vi "deleteDetails.vi"(8 "error in (no error)":errorcluster, 10 "details":T2, 11 "reference in":refnum<class "Devices Controller.lvclass">) -> (0 "error out":errorcluster, 3 "reference out":refnum<class "Devices Controller.lvclass">)   [LabVIEW 2015, in "Devices Controller.lvclass"]
uses:
  Devices Controller.lvclass
  deviceType.ctl
  APP/excelFile_class/fileType.ctl
  APP/k4b2_class/k4b2.lvclass
  APP/fitmate_class/fitmate.lvclass
  APP/cpet_class/cpet.lvclass
  APP/rmr_class/rmr.lvclass
  APP/bb-pft_class/bb-pft.lvclass
  APP/bodpod_class/bodpod.lvclass
  APP/peapod_class/peapod.lvclass
  APP/k5_class/k5.lvclass
  APP/excelFile_class/excelFile.lvclass
  File Controller_llb/File Controller.lvclass
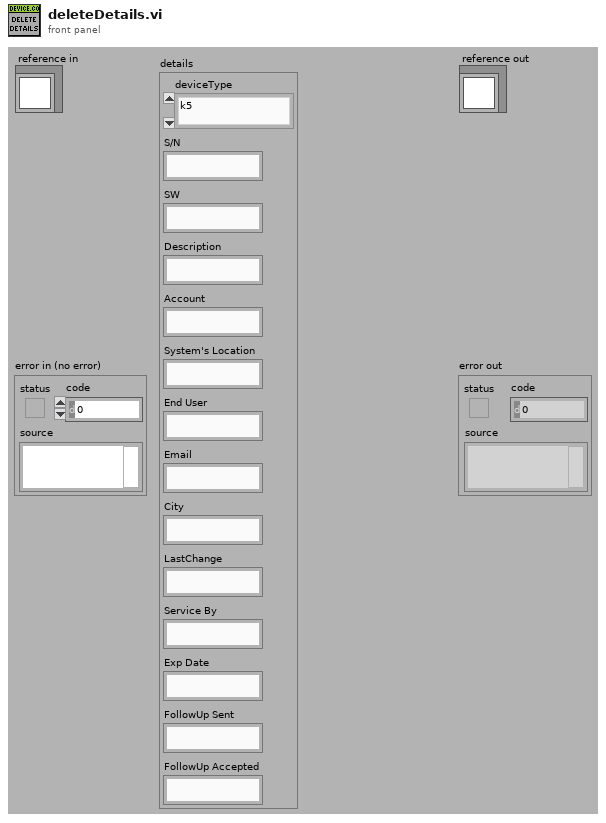
[diagram p1: front panel]
types:
  T1 = typedef "Devices Controller.lvclass/deviceType.ctl" = enum16{"k5", "k4b2", "fitmate", "cpet", "rmr", "bodyBoxPft", "bp", "pp"}
  T2 = cluster{"deviceType":T1, "S/N":string, "SW":string, "Description":string, "Account":string, "System's Location":string, "End User":string, "Email":string, "City":string, "LastChange":string, "Service By":string, "Exp Date":string, "FollowUp Sent":string, "FollowUp Accepted":string}
  T3 = typedef "excelFile.lvclass/fileType.ctl" = enum16{"devices", "items", "partsTracking", "TSR"}
  T4 = typedef "Devices Controller.lvclass/ObjectAttributesRef.ctl" = refnum<data-value>
  T5 = typedef "Devices Controller.lvclass/ObjectAttributes.ctl" = cluster{"MyAttribute":dbl, "file_controller_ref":refnum<class "File Controller.lvclass">, "data":string[][][], "devices_refs":cluster{"k4b2_refs":refnum<class "k4b2.lvclass">[], "rmr_refs":refnum<class "rmr.lvclass">[], "bod_pod_refs":refnum<class "bodpod.lvclass">[], "cpet_refs":refnum<class "cpet.lvclass">[], "fitmate_refs":refnum<class "fitmate.lvclass">[], "pea_pod_refs":refnum<class "peapod.lvclass">[], "k5_refs":refnum<class "k5.lvclass">[], "bb-pft_refs":refnum<class "bb-pft.lvclass">[]}}
  T6 = cluster{"k4b2_refs":refnum<class "k4b2.lvclass">[], "rmr_refs":refnum<class "rmr.lvclass">[], "bod_pod_refs":refnum<class "bodpod.lvclass">[], "cpet_refs":refnum<class "cpet.lvclass">[], "fitmate_refs":refnum<class "fitmate.lvclass">[], "pea_pod_refs":refnum<class "peapod.lvclass">[], "k5_refs":refnum<class "k5.lvclass">[], "bb-pft_refs":refnum<class "bb-pft.lvclass">[]}
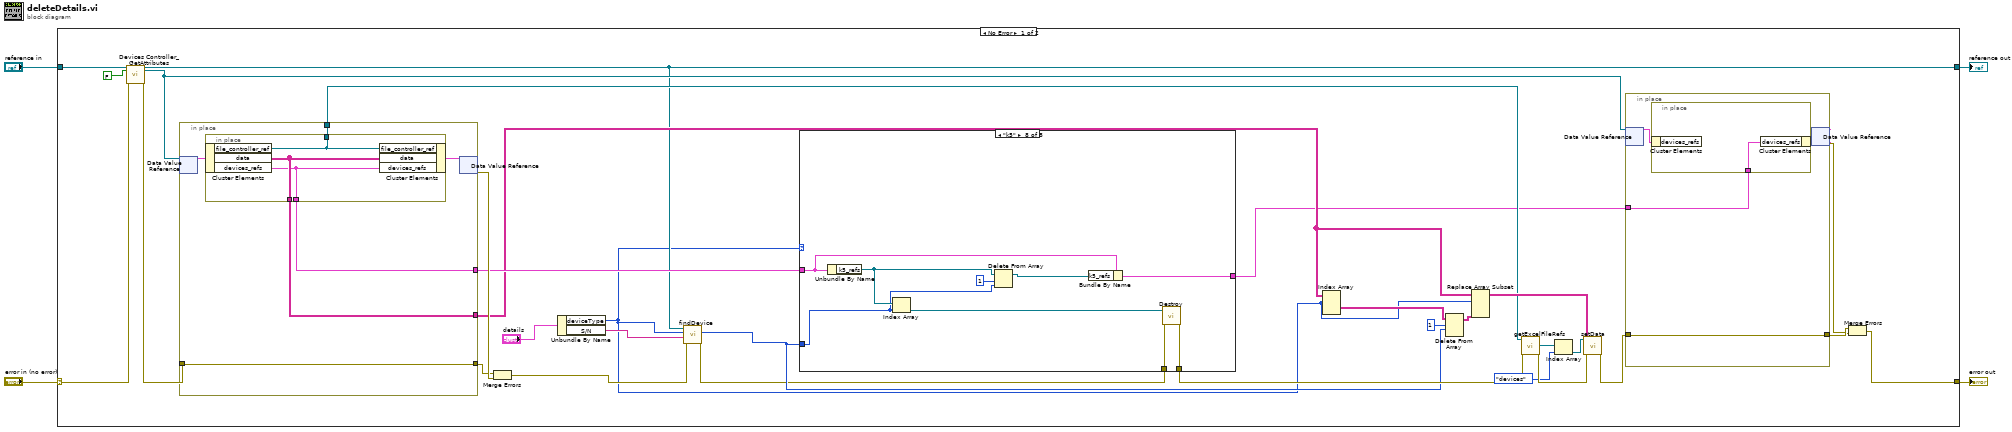
[diagram p0: block diagram]
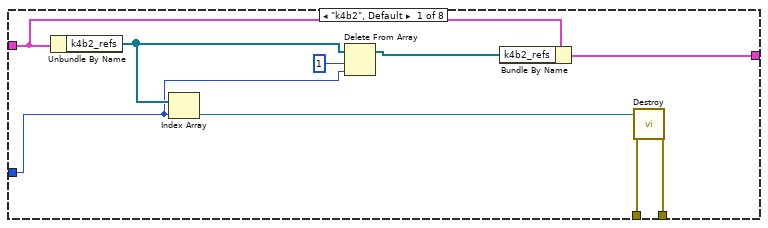
[diagram p2: hidden frame]
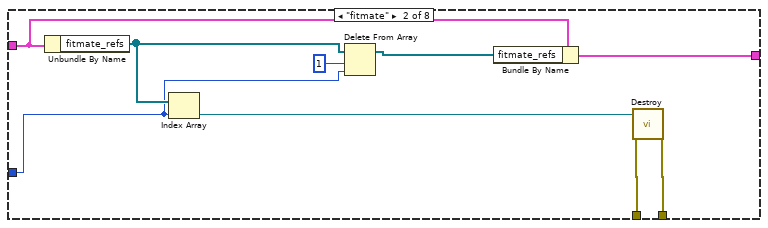
[diagram p3: hidden frame]
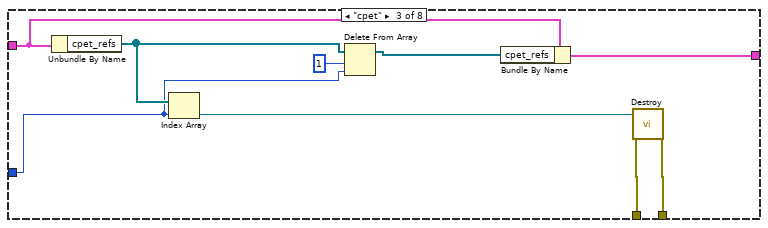
[diagram p4: hidden frame]
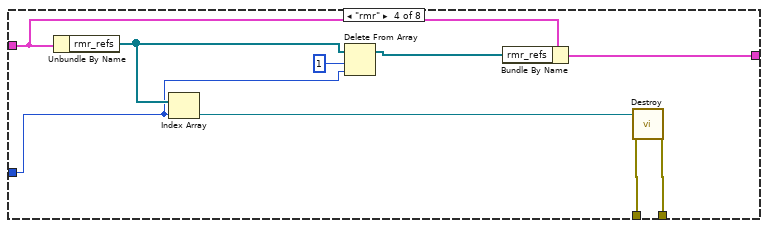
[diagram p5: hidden frame]
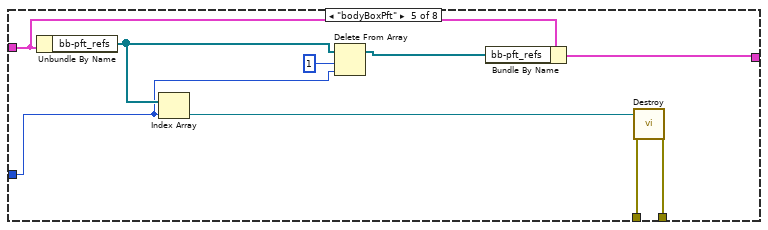
[diagram p6: hidden frame]
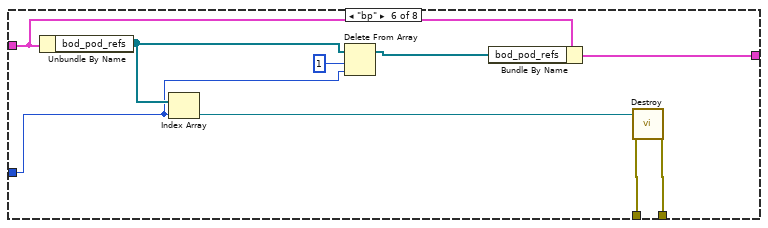
[diagram p7: hidden frame]
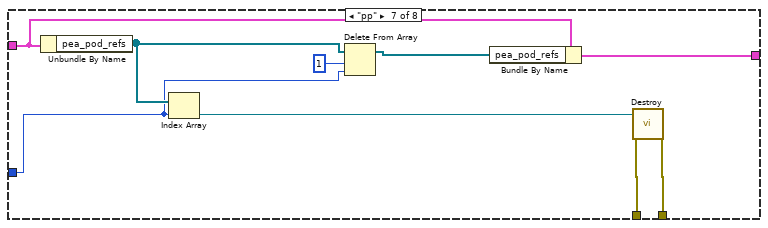
[diagram p8: hidden frame]
diagram:
  n1 = case shown="No Error" "error in (no error)" {
    selector: "error in (no error)" -> [w31 w123]
    tunnel: [w11 w123] -> w3
    tunnel: [w10 w122] -> w1
    tunnel: "reference in" -> [w33 w122]
    frame No Error {
      n2 = call "Devices Controller_GetAttributes.vi"("reference in"=w33, "return data? (T)"=FALSE, "error in (no error)"=w31) -> ("reference out"=w10:refnum<class "Devices Controller.lvclass">, "attributes ref"=w14:T4, "error out"=w30:errorcluster)  [unwired: 13 in, 1 out]
      n3 = in-place {
        in-place-border: w30 -> [w116]
        in-place-border: [w116] -> w34
        in-place-border: [w115] -> w20
        in-place-border: [w114] -> w29
        in-place-border: [w113] -> w19
        n4 = in-place-dvr #1(w14) -> (w117:T5)  [unwired: 1 out]
        n5 = in-place {
          in-place-border: [w121] -> w115
          in-place-border: [w120] -> w114
          in-place-border: [w119] -> w113
          n6 = in-place-cluster #2(w117) -> ("file_controller_ref"=w119:refnum<class "File Controller.lvclass">, "data"=w121:string[][][], "devices_refs"=w120:T6)
          n7 = in-place-cluster #2("file_controller_ref"=w119, "data"=w121, "devices_refs"=w120) -> (w118:T5)
        }
        n8 = in-place-dvr #1(w118) -> (w35:errorcluster)  [unwired: 1 out]
      }
      n9 = Merge Errors(w34, w35) -> (w8:errorcluster)
      n10 = Unbundle By Name("details") -> ("deviceType"=w5:T1, "S/N"=w6:string)
      n11 = call "findDevice.vi"("error in (no error)"=w8, "S/N:"=w6, "Device Type:"=w5, "reference in"=w10) -> ("error out"=w7:errorcluster, "index of element"=w9:i32)  [unwired: 4 in, 2 out]
      n12 = case shown="\"k5\"" w5 {
        tunnel: w29 -> [w43 w52 w61 w70 w81 w88 w97 w109]
        tunnel: w9 -> [w44 w53 w62 w71 w80 w89 w98 w108]
        tunnel: w7 -> [w49 w58 w67 w76 w78 w94 w103 w105]
        tunnel: [w48 w57 w66 w75 w77 w93 w102 w104] -> w21
        tunnel: [w41 w50 w59 w68 w79 w86 w95 w106] -> w15
        frame "k4b2", Default {
          n13 = Unbundle By Name(w43) -> ("k4b2_refs"=w45:refnum<class "k4b2.lvclass">[])
          n14 = Index Array(array=w45, index=w44) -> (element=w47:refnum<class "k4b2.lvclass">)
          n15 = Delete From Array(array=w45, length=1, index=w44) -> (array with subset deleted=w42:refnum<class "k4b2.lvclass">[])  [unwired: 1 out]
          n16 = Bundle By Name(cluster=w43, "k4b2_refs"=w42) -> (w41:T6)
          n17 = call-dynamic "Destroy.vi"("reference in"=w47, "error in (no error)"=w49) -> ("error out"=w48:errorcluster)  [unwired: 16 in, 1 out]
        }
        frame "fitmate" {
          n18 = Unbundle By Name(w52) -> ("fitmate_refs"=w54:refnum<class "fitmate.lvclass">[])
          n19 = Index Array(array=w54, index=w53) -> (element=w56:refnum<class "fitmate.lvclass">)
          n20 = Delete From Array(array=w54, length=1, index=w53) -> (array with subset deleted=w51:refnum<class "fitmate.lvclass">[])  [unwired: 1 out]
          n21 = Bundle By Name(cluster=w52, "fitmate_refs"=w51) -> (w50:T6)
          n22 = call-dynamic "Destroy.vi"("reference in"=w56, "error in (no error)"=w58) -> ("error out"=w57:errorcluster)  [unwired: 16 in, 1 out]
        }
        frame "cpet" {
          n23 = Unbundle By Name(w61) -> ("cpet_refs"=w63:refnum<class "cpet.lvclass">[])
          n24 = Index Array(array=w63, index=w62) -> (element=w65:refnum<class "cpet.lvclass">)
          n25 = Delete From Array(array=w63, length=1, index=w62) -> (array with subset deleted=w60:refnum<class "cpet.lvclass">[])  [unwired: 1 out]
          n26 = Bundle By Name(cluster=w61, "cpet_refs"=w60) -> (w59:T6)
          n27 = call-dynamic "Destroy.vi"("reference in"=w65, "error in (no error)"=w67) -> ("error out"=w66:errorcluster)  [unwired: 16 in, 1 out]
        }
        frame "rmr" {
          n28 = Unbundle By Name(w70) -> ("rmr_refs"=w72:refnum<class "rmr.lvclass">[])
          n29 = Index Array(array=w72, index=w71) -> (element=w74:refnum<class "rmr.lvclass">)
          n30 = Delete From Array(array=w72, length=1, index=w71) -> (array with subset deleted=w69:refnum<class "rmr.lvclass">[])  [unwired: 1 out]
          n31 = Bundle By Name(cluster=w70, "rmr_refs"=w69) -> (w68:T6)
          n32 = call-dynamic "Destroy.vi"("reference in"=w74, "error in (no error)"=w76) -> ("error out"=w75:errorcluster)  [unwired: 16 in, 1 out]
        }
        frame "bodyBoxPft" {
          n33 = Unbundle By Name(w81) -> ("bb-pft_refs"=w83:refnum<class "bb-pft.lvclass">[])
          n34 = Index Array(array=w83, index=w80) -> (element=w85:refnum<class "bb-pft.lvclass">)
          n35 = Delete From Array(array=w83, length=1, index=w80) -> (array with subset deleted=w82:refnum<class "bb-pft.lvclass">[])  [unwired: 1 out]
          n36 = Bundle By Name(cluster=w81, "bb-pft_refs"=w82) -> (w79:T6)
          n37 = call-dynamic "Destroy.vi"("reference in"=w85, "error in (no error)"=w78) -> ("error out"=w77:errorcluster)  [unwired: 16 in, 1 out]
        }
        frame "bp" {
          n38 = Unbundle By Name(w88) -> ("bod_pod_refs"=w90:refnum<class "bodpod.lvclass">[])
          n39 = Index Array(array=w90, index=w89) -> (element=w92:refnum<class "bodpod.lvclass">)
          n40 = Delete From Array(array=w90, length=1, index=w89) -> (array with subset deleted=w87:refnum<class "bodpod.lvclass">[])  [unwired: 1 out]
          n41 = Bundle By Name(cluster=w88, "bod_pod_refs"=w87) -> (w86:T6)
          n42 = call-dynamic "Destroy.vi"("reference in"=w92, "error in (no error)"=w94) -> ("error out"=w93:errorcluster)  [unwired: 16 in, 1 out]
        }
        frame "pp" {
          n43 = Unbundle By Name(w97) -> ("pea_pod_refs"=w99:refnum<class "peapod.lvclass">[])
          n44 = Index Array(array=w99, index=w98) -> (element=w101:refnum<class "peapod.lvclass">)
          n45 = Delete From Array(array=w99, length=1, index=w98) -> (array with subset deleted=w96:refnum<class "peapod.lvclass">[])  [unwired: 1 out]
          n46 = Bundle By Name(cluster=w97, "pea_pod_refs"=w96) -> (w95:T6)
          n47 = call-dynamic "Destroy.vi"("reference in"=w101, "error in (no error)"=w103) -> ("error out"=w102:errorcluster)  [unwired: 16 in, 1 out]
        }
        frame "k5" {
          n48 = Unbundle By Name(w109) -> ("k5_refs"=w110:refnum<class "k5.lvclass">[])
          n49 = Index Array(array=w110, index=w108) -> (element=w112:refnum<class "k5.lvclass">)
          n50 = Delete From Array(array=w110, length=1, index=w108) -> (array with subset deleted=w107:refnum<class "k5.lvclass">[])  [unwired: 1 out]
          n51 = Bundle By Name(cluster=w109, "k5_refs"=w107) -> (w106:T6)
          n52 = call-dynamic "Destroy.vi"("reference in"=w112, "error in (no error)"=w105) -> ("error out"=w104:errorcluster)  [unwired: 16 in, 1 out]
        }
      }
      n53 = Index Array(array=w20, index (dim 0)=w5) -> (element=w28:string[][])  [unwired: 2 in]
      n54 = Delete From Array(array=w28, length=1, index (row)=w9) -> (array with subset deleted=w27:string[][])  [unwired: 1 in, 1 out]
      n55 = Replace Array Subset(array=w20, new element=w27, index (dim 0)=w5) -> (w26:string[][][])  [unwired: 2 in]
      n56 = call "getExcelFileRefs.vi"("error in (no error)"=w21, "reference in"=w19) -> ("error out"=w25:errorcluster, "excelFile_refs"=w24:refnum<class "excelFile.lvclass">[])  [unwired: 7 in, 1 out]
      n57 = Index Array(array=w24, index=fileType."devices" ("fileType")) -> (element=w23:refnum<class "excelFile.lvclass">)
      n58 = call "setData.vi"("error in (no error)"=w25, "data"=w26, "reference in"=w23) -> ("error out"=w16:errorcluster)  [unwired: 7 in, 1 out]
      n59 = in-place {
        in-place-border: w16 -> [w37]
        in-place-border: [w37] -> w13
        in-place-border: w15 -> [w36]
        n60 = in-place-dvr #3(w14) -> (w38:T5)  [unwired: 1 out]
        n61 = in-place {
          in-place-border: w36 -> [w40]
          n62 = in-place-cluster #4(w38) -> ()  [unwired: 1 out]
          n63 = in-place-cluster #4("devices_refs"=w40) -> (w39:T5)
        }
        n64 = in-place-dvr #3(w39) -> (w12:errorcluster)  [unwired: 1 out]
      }
      n65 = Merge Errors(w13, w12) -> (w11:errorcluster)
    }
    frame Error {
    }
  }
  "error out" <- w3
  "reference out" <- w1
